vi "GeoData.vi"() -> ()   [LabVIEW 2017] (continued)
H1\n16631\t42013\tCurryville\tPA\tBlair County\tH1\n16870\t42013\tPort matilda\tPA\tBlair County\tH1\n16635\t42013\tDuncansville\tPA\tBlair County\tH1\n16613\t42013\tAshville\tPA\tBlair County\tH1\n16686\t42013\tTyrone\tPA\tBlair County\tH1\n16602\t42013\tAltoona\tPA\tBlair County\tH1\n16673\t42013\tRoaring spring\tPA\tBlair County\tH1\n16662\t42013\tMartinsburg\tPA\tBlair County\tH1\n16682\t42013\tSproul\tPA\tBlair County\tH1\n18616\t42015\tForksville\tPA\tBradford County\tH1\n18837\t42015\tRome\tPA\tBradford County\tH1\n18846\t42015\tSugar run\tPA\tBradford County\tH1\n16914\t42015\tColumbia cross roads\tPA\tBradford County\tH1\n18832\t42015\tMonroeton\tPA\tBradford County\tH1\n17765\t42015\tRoaring branch\tPA\tBradford County\tH1\n18623\t42015\tLaceyville\tPA\tBradford County\tH1\n18810\t42015\tAthens\tPA\tBradford County\tH1\n18833\t42015\tNew albany\tPA\tBradford County\tH1\n18830\t42015\tLittle meadows\tPA\tBradford County\tH1\n16926\t42015\tGranville summit\tPA\tBradford County\tH1\n18817\t42015\tEast smithfield\tPA\tBradford County\tH1\n16925\t42015\tGillett\tPA\tBradford County\tH1\n18840\t42015\tSayre\tPA\tBradford County\tH1\n18850\t42015\tUlster\tPA\tBradford County\tH1\n18814\t42015\tBurlington\tPA\tBradford County\tH1\n17735\t42015\tGrover\tPA\tBradford County\tH1\n18853\t42015\tWyalusing\tPA\tBradford County\tH1\n18854\t42015\tWysox\tPA\tBradford County\tH1\n18848\t42015\tTowanda\tPA\tBradford County\tH1\n18851\t42015\tWarren center\tPA\tBradford County\tH1\n18831\t42015\tMilan\tPA\tBradford County\tH1\n17724\t42015\tCanton\tPA\tBradford County\tH1\n18845\t42015\tStevensville\tPA\tBradford County\tH1\n16910\t42015\tAlba\tPA\tBradford County\tH1\n16936\t42015\tMillerton\tPA\tBradford County\tH1\n16947\t42015\tTroy\tPA\tBradford County\tH1\n18614\t42015\tDushore\tPA\tBradford County\tH1\n18829\t42015\tLe raysville\tPA\tBradford County\tH1\n16945\t42015\tSylvania\tPA\tBradford County\tH1\n18930\t42017\tKintnersville\tPA\tBucks County\tH1\n19006\t42017\tHuntingdon valley\tPA\tBucks County\tH1\n19047\t42017\tLanghorne\tPA\tBucks County\tH1\n19055\t42017\tLevittown\tPA\tBucks County\tH1\n18081\t42017\tSpringtown\tPA\tBucks County\tH1\n18970\t42017\tTrumbauersville\tPA\tBucks County\tH1\n18917\t42017\tDublin\tPA\tBucks County\tH1\n18931\t42017\tLahaska\tPA\tBucks County\tH1\n18968\t42017\tSpinnerstown\tPA\tBucks County\tH1\n18956\t42017\tRushland\tPA\tBucks County\tH1\n18925\t42017\tFurlong\tPA\tBucks County\tH1\n18972\t42017\tUpper black eddy\tPA\tBucks County\tH1\n19030\t42017\tFairless hills\tPA\tBucks County\tH1\n19057\t42017\tLevittown\tPA\tBucks County\tH1\n18055\t42017\tHellertown\tPA\tBucks County\tH1\n18914\t42017\tChalfont\tPA\tBucks County\tH1\n18912\t42017\tBuckingham\tPA\tBucks County\tH1\n18951\t42017\tQuakertown\tPA\tBucks County\tH1\n18964\t42017\tSouderton\tPA\tBucks County\tH1\n18942\t42017\tOttsville\tPA\tBucks County\tH1\n18977\t42017\tWashington crossing\tPA\tBucks County\tH1\n19044\t42017\tHorsham\tPA\tBucks County\tH1\n19440\t42017\tHatfield\tPA\tBucks County\tH1\n18935\t42017\tMilford square\tPA\tBucks County\tH1\n18981\t42017\tZionhill\tPA\tBucks County\tH1\n18946\t42017\tPineville\tPA\tBucks County\tH1\n18036\t42017\tCoopersburg\tPA\tBucks County\tH1\n18041\t42017\tEast greenville\tPA\tBucks County\tH1\n18077\t42017\tRiegelsville\tPA\tBucks County\tH1\n18954\t42017\tRichboro\tPA\tBucks County\tH1\n18940\t42017\tNewtown\tPA\tBucks County\tH1\n19007\t42017\tBristol\tPA\tBucks County\tH1\n19454\t42017\tNorth wales\tPA\tBucks County\tH1\n18934\t42017\tMechanicsville\tPA\tBucks County\tH1\n18933\t42017\tLumberville\tPA\tBucks County\tH1\n18915\t42017\tColmar\tPA\tBucks County\tH1\n19067\t42017\tMorrisville\tPA\tBucks County\tH1\n19053\t42017\tFeasterville trevose\tPA\tBucks County\tH1\n18949\t42017\tPlumsteadville\tPA\tBucks County\tH1\n18963\t42017\tSolebury\tPA\tBucks County\tH1\n18928\t42017\tHolicong\tPA\tBucks County\tH1\n18913\t42017\tCarversville\tPA\tBucks County\tH1\n18943\t42017\tPenns park\tPA\tBucks County\tH1\n18042\t42017\tEaston\tPA\tBucks County\tH1\n18054\t42017\tGreen lane\tPA\tBucks County\tH1\n18938\t42017\tNew hope\tPA\tBucks County\tH1\n18901\t42017\tDoylestown\tPA\tBucks County\tH1\n18929\t42017\tJamison\tPA\tBucks County\tH1\n18923\t42017\tFountainville\tPA\tBucks County\tH1\n18932\t42017\tLine lexington\tPA\tBucks County\tH1\n18974\t42017\tWarminster\tPA\tBucks County\tH1\n18960\t42017\tSellersville\tPA\tBucks County\tH1\n18976\t42017\tWarrington\tPA\tBucks County\tH1\n18947\t42017\tPipersville\tPA\tBucks County\tH1\n18962\t42017\tSilverdale\tPA\tBucks County\tH1\n19020\t42017\tBensalem\tPA\tBucks County\tH1\n19021\t42017\tCroydon\tPA\tBucks County\tH1\n19040\t42017\tHatboro\tPA\tBucks County\tH1\n18953\t42017\tRevere\tPA\tBucks County\tH1\n18911\t42017\tBlooming glen\tPA\tBucks County\tH1\n18073\t42017\tPennsburg\tPA\tBucks County\tH1\n18902\t42017\tDoylestown\tPA\tBucks County\tH1\n19056\t42017\tLevittown\tPA\tBucks County\tH1\n19058\t42017\tLevittown\tPA\tBucks County\tH1\n19054\t42017\tLevittown\tPA\tBucks County\tH1\n18955\t42017\tRichlandtown\tPA\tBucks County\tH1\n18950\t42017\tPoint pleasant\tPA\tBucks County\tH1\n18980\t42017\tWycombe\tPA\tBucks County\tH1\n18039\t42017\tDurham\tPA\tBucks County\tH1\n18944\t42017\tPerkasie\tPA\tBucks County\tH1\n18966\t42017\tSouthampton\tPA\tBucks County\tH1\n18969\t42017\tTelford\tPA\tBucks County\tH1\n18927\t42017\tHilltown\tPA\tBucks County\tH1\n18920\t42017\tErwinna\tPA\tBucks County\tH1\n18922\t42017\tForest grove\tPA\tBucks County\tH1\n18910\t42017\tBedminster\tPA\tBucks County\tH1\n18916\t42017\tDanboro\tPA\tBucks County\tH1\n18921\t42017\tFerndale\tPA\tBucks County\tH1\n16001\t42019\tButler\tPA\tButler County\tH1\n16051\t42019\tPortersville\tPA\tButler County\tH1\n16127\t42019\tGrove city\tPA\tButler County\tH1\n16059\t42019\tValencia\tPA\tButler County\tH1\n16053\t42019\tRenfrew\tPA\tButler County\tH1\n16052\t42019\tProspect\tPA\tButler County\tH1\n16041\t42019\tKarns city\tPA\tButler County\tH1\n16030\t42019\tEau claire\tPA\tButler County\tH1\n16035\t42019\tForestville\tPA\tButler County\tH1\n16024\t42019\tCallery\tPA\tButler County\tH1\n15044\t42019\tGibsonia\tPA\tButler County\tH1\n16002\t42019\tButler\tPA\tButler County\tH1\n16049\t42019\tParker\tPA\tButler County\tH1\n16038\t42019\tHarrisville\tPA\tButler County\tH1\n16040\t42019\tHilliards\tPA\tButler County\tH1\n16063\t42019\tZelienople\tPA\tButler County\tH1\n16066\t42019\tCranberry township\tPA\tButler County\tH1\n16034\t42019\tFenelton\tPA\tButler County\tH1\n16048\t42019\tNorth washington\tPA\tButler County\tH1\n16033\t42019\tEvans city\tPA\tButler County\tH1\n16373\t42019\tEmlenton\tPA\tButler County\tH1\n16050\t42019\tPetrolia\tPA\tButler County\tH1\n16029\t42019\tEast butler\tPA\tButler County\tH1\n16022\t42019\tBruin\tPA\tButler County\tH1\n16025\t42019\tChicora\tPA\tButler County\tH1\n15086\t42019\tWarrendale\tPA\tButler County\tH1\n16020\t42019\tBoyers\tPA\tButler County\tH1\n16039\t42019\tHerman\tPA\tButler County\tH1\n15065\t42019\tNatrona heights\tPA\tButler County\tH1\n16045\t42019\tLyndora\tPA\tButler County\tH1\n16023\t42019\tCabot\tPA\tButler County\tH1\n16027\t42019\tConnoquenessing\tPA\tButler County\tH1\n16046\t42019\tMars\tPA\tButler County\tH1\n16061\t42019\tWest sunbury\tPA\tButler County\tH1\n16003\t42019\tButler\tPA\tButler County\tH1\n16056\t42019\tSaxonburg\tPA\tButler County\tH1\n16057\t42019\tSlippery rock\tPA\tButler County\tH1\n16055\t42019\tSarver\tPA\tButler County\tH1\n16037\t42019\tHarmony\tPA\tButler County\tH1\n16229\t42019\tFreeport\tPA\tButler County\tH1\n15906\t42021\tJohnstown\tPA\tCambria County\tH1\n15901\t42021\tJohnstown\tPA\tCambria County\tH1\n15958\t42021\tSummerhill\tPA\tCambria County\tH1\n16639\t42021\tFallentimber\tPA\tCambria County\tH1\n15762\t42021\tNicktown\tPA\tCambria County\tH1\n15738\t42021\tEmeigh\tPA\tCambria County\tH1\n15934\t42021\tElton\tPA\tCambria County\tH1\n15930\t42021\tDunlo\tPA\tCambria County\tH1\n15714\t42021\tNorthern cambria\tPA\tCambria County\tH1\n15946\t42021\tPortage\tPA\tCambria County\tH1\n15955\t42021\tSidman\tPA\tCambria County\tH1\n16601\t42021\tAltoona\tPA\tCambria County\tH1\n15760\t42021\tMarsteller\tPA\tCambria County\tH1\n15956\t42021\tSouth fork\tPA\tCambria County\tH1\n16629\t42021\tCoupon\tPA\tCambria County\tH1\n15922\t42021\tBelsano\tPA\tCambria County\tH1\n15962\t42021\tWilmore\tPA\tCambria County\tH1\n15938\t42021\tLilly\tPA\tCambria County\tH1\n15902\t42021\tJohnstown\tPA\tCambria County\tH1\n15931\t42021\tEbensburg\tPA\tCambria County\tH1\n15940\t42021\tLoretto\tPA\tCambria County\tH1\n15957\t42021\tStrongstown\tPA\tCambria County\tH1\n16636\t42021\tDysart\tPA\tCambria County\tH1\n15927\t42021\tColver\tPA\tCambria County\tH1\n15773\t42021\tSaint benedict\tPA\tCambria County\tH1\n15904\t42021\tJohnstown\tPA\tCambria County\tH1\n15952\t42021\tSalix\tPA\tCambria County\tH1\n16641\t42021\tGallitzin\tPA\tCambria County\tH1\n16627\t42021\tCoalport\tPA\tCambria County\tH1\n16640\t42021\tFlinton\tPA\tCambria County\tH1\n16646\t42021\tHastings\tPA\tCambria County\tH1\n15961\t42021\tVintondale\tPA\tCambria County\tH1\n15921\t42021\tBeaverdale\tPA\tCambria County\tH1\n15951\t42021\tSaint michael\tPA\tCambria County\tH1\n15948\t42021\tRevloc\tPA\tCambria County\tH1\n15960\t42021\tTwin rocks\tPA\tCambria County\tH1\n15915\t42021\tJohnstown\tPA\tCambria County\tH1\n15724\t42021\tCherry tree\tPA\tCambria County\tH1\n15909\t42021\tJohnstown\tPA\tCambria County\tH1\n15943\t42021\tNanty glo\tPA\tCambria County\tH1\n15963\t42021\tWindber\tPA\tCambria County\tH1\n15722\t42021\tCarrolltown\tPA\tCambria County\tH1\n16675\t42021\tSaint boniface\tPA\tCambria County\tH1\n16624\t42021\tChest springs\tPA\tCambria County\tH1\n15907\t42021\tJohnstown\tPA\tCambria County\tH1\n16635\t42021\tDuncansville\tPA\tCambria County\tH1\n16613\t42021\tAshville\tPA\tCambria County\tH1\n16619\t42021\tBlandburg\tPA\tCambria County\tH1\n15775\t42021\tSpangler\tPA\tCambria County\tH1\n15905\t42021\tJohnstown\tPA\tCambria County\tH1\n15942\t42021\tMineral point\tPA\tCambria County\tH1\n16630\t42021\tCresson\tPA\tCambria County\tH1\n16668\t42021\tPatton\tPA\tCambria County\tH1\n15959\t42021\tTire hill\tPA\tCambria County\tH1\n15945\t42021\tParkhill\tPA\tCambria County\tH1\n15737\t42021\tElmora\tPA\tCambria County\tH1\n16644\t42021\tGlasgow\tPA\tCambria County\tH1\n15925\t42021\tCassandra\tPA\tCambria County\tH1\n15832\t42023\tDriftwood\tPA\tCameron County\tH1\n15861\t42023\tSinnamahoning\tPA\tCameron County\tH1\n16720\t42023\tAustin\tPA\tCameron County\tH1\n15834\t42023\tEmporium\tPA\tCameron County\tH1\n18211\t42025\tAndreas\tPA\tCarbon County\tH1\n18252\t42025\tTamaqua\tPA\tCarbon County\tH1\n18012\t42025\tAquashicola\tPA\tCarbon County\tH1\n18229\t42025\tJim thorpe\tPA\tCarbon County\tH1\n18254\t42025\tTresckow\tPA\tCarbon County\tH1\n18661\t42025\tWhite haven\tPA\tCarbon County\tH1\n18624\t42025\tLake harmony\tPA\tCarbon County\tH1\n18030\t42025\tBowmanstown\tPA\tCarbon County\tH1\n18053\t42025\tGermansville\tPA\tCarbon County\tH1\n18240\t42025\tNesquehoning\tPA\tCarbon County\tH1\n18333\t42025\tKresgeville\tPA\tCarbon County\tH1\n18230\t42025\tJunedale\tPA\tCarbon County\tH1\n18071\t42025\tPalmerton\tPA\tCarbon County\tH1\n18250\t42025\tSummit hill\tPA\tCarbon County\tH1\n18216\t42025\tBeaver meadows\tPA\tCarbon County\tH1\n18212\t42025\tAshfield\tPA\tCarbon County\tH1\n18232\t42025\tLansford\tPA\tCarbon County\tH1\n18244\t42025\tParryville\tPA\tCarbon County\tH1\n18201\t42025\tHazleton\tPA\tCarbon County\tH1\n18235\t42025\tLehighton\tPA\tCarbon County\tH1\n18255\t42025\tWeatherly\tPA\tCarbon County\tH1\n18237\t42025\tMcadoo\tPA\tCarbon County\tH1\n18058\t42025\tKunkletown\tPA\tCarbon County\tH1\n18210\t42025\tAlbrightsville\tPA\tCarbon County\tH1\n16820\t42027\tAaronsburg\tPA\tCentre County\tH1\n16829\t42027\tClarence\tPA\tCentre County\tH1\n16677\t42027\tSandy ridge\tPA\tCentre County\tH1\n16666\t42027\tOsceola mills\tPA\tCentre County\tH1\n16865\t42027\tPennsylvania furnace\tPA\tCentre County\tH1\n16844\t42027\tJulian\tPA\tCentre County\tH1\n16801\t42027\tState college\tPA\tCentre County\tH1\n16823\t42027\tBellefonte\tPA\tCentre County\tH1\n16866\t42027\tPhilipsburg\tPA\tCentre County\tH1\n16854\t42027\tMillheim\tPA\tCentre County\tH1\n16826\t42027\tBlanchard\tPA\tCentre County\tH1\n16804\t42027\tState college\tPA\tCentre County\tH1\n16853\t42027\tMilesburg\tPA\tCentre County\tH1\n16835\t42027\tFleming\tPA\tCentre County\tH1\n16803\t42027\tState college\tPA\tCentre County\tH1\n16827\t42027\tBoalsburg\tPA\tCentre County\tH1\n16870\t42027\tPort matilda\tPA\tCentre County\tH1\n16802\t42027\tUniversity park\tPA\tCentre County\tH1\n16872\t42027\tRebersburg\tPA\tCentre County\tH1\n16852\t42027\tMadisonburg\tPA\tCentre County\tH1\n16860\t42027\tMunson\tPA\tCentre County\tH1\n16868\t42027\tPine grove mills\tPA\tCentre County\tH1\n16856\t42027\tMingoville\tPA\tCentre County\tH1\n16686\t42027\tTyrone\tPA\tCentre County\tH1\n16828\t42027\tCentre hall\tPA\tCentre County\tH1\n16822\t42027\tBeech creek\tPA\tCentre County\tH1\n16874\t42027\tSnow shoe\tPA\tCentre County\tH1\n16845\t42027\tKarthaus\tPA\tCentre County\tH1\n16859\t42027\tMoshannon\tPA\tCentre County\tH1\n16877\t42027\tWarriors mark\tPA\tCentre County\tH1\n16851\t42027\tLemont\tPA\tCentre County\tH1\n16841\t42027\tHoward\tPA\tCentre County\tH1\n16875\t42027\tSpring mills\tPA\tCentre County\tH1\n16882\t42027\tWoodward\tPA\tCentre County\tH1\n16832\t42027\tCoburn\tPA\tCentre County\tH1\n16864\t42027\tOrviston\tPA\tCentre County\tH1\n19355\t42029\tMalvern\tPA\tChester County\tH1\n19311\t42029\tAvondale\tPA\tChester County\tH1\n19363\t42029\tOxford\tPA\tChester County\tH1\n19465\t42029\tPottstown\tPA\tChester County\tH1\n19480\t42029\tUwchland\tPA\tChester County\tH1\n19481\t42029\tValley forge\tPA\tChester County\tH1\n19357\t42029\tMendenhall\tPA\tChester County\tH1\n19432\t42029\tDevault\tPA\tChester County\tH1\n19367\t42029\tPomeroy\tPA\tChester County\tH1\n19365\t42029\tParkesburg\tPA\tChester County\tH1\n19425\t42029\tChester springs\tPA\tChester County\tH1\n19475\t42029\tSpring city\tPA\tChester County\tH1\n17536\t42029\tKirkwood\tPA\tChester County\tH1\n19354\t42029\tLyndell\tPA\tChester County\tH1\n17555\t42029\tNarvon\tPA\tChester County\tH1\n19073\t42029\tNewtown square\tPA\tChester County\tH1\n19330\t42029\tCochranville\tPA\tChester County\tH1\n19341\t42029\tExton\tPA\tChester County\tH1\n19317\t42029\tChadds ford\tPA\tChester County\tH1\n19372\t42029\tThorndale\tPA\tChester County\tH1\n19543\t42029\tMorgantown\tPA\tChester County\tH1\n19399\t42029\tSoutheastern\tPA\tChester County\tH1\n19319\t42029\tCheyney\tPA\tChester County\tH1\n19421\t42029\tBirchrunville\tPA\tChester County\tH1\n19371\t42029\tSuplee\tPA\tChester County\tH1\n17527\t42029\tGap\tPA\tChester County\tH1\n19352\t42029\tLincoln university\tPA\tChester County\tH1\n19395\t42029\tWesttown\tPA\tChester County\tH1\n19381\t42029\tWest chester\tPA\tChester County\tH1\n19460\t42029\tPhoenixville\tPA\tChester County\tH1\n19351\t42029\tLewisville\tPA\tChester County\tH1\n19347\t42029\tKemblesville\tPA\tChester County\tH1\n19366\t42029\tPocopson\tPA\tChester County\tH1\n19520\t42029\tElverson\tPA\tChester County\tH1\n19350\t42029\tLandenberg\tPA\tChester County\tH1\n19335\t42029\tDowningtown\tPA\tChester County\tH1\n19344\t42029\tHoney brook\tPA\tChester County\tH1\n19382\t42029\tWest chester\tPA\tChester County\tH1\n19464\t42029\tPottstown\tPA\tChester County\tH1\n19375\t42029\tUnionville\tPA\tChester County\tH1\n19470\t42029\tSaint peters\tPA\tChester County\tH1\n19087\t42029\tWayne\tPA\tChester County\tH1\n19348\t42029\tKennett square\tPA\tChester County\tH1\n19380\t42029\tWest chester\tPA\tChester County\tH1\n19390\t42029\tWest grove\tPA\tChester County\tH1\n19376\t42029\tWagontown\tPA\tChester County\tH1\n19316\t42029\tBrandamore\tPA\tChester County\tH1\n19320\t42029\tCoatesville\tPA\tChester County\tH1\n19333\t42029\tDevon\tPA\tChester County\tH1\n19343\t42029\tGlenmoore\tPA\tChester County\tH1\n19442\t42029\tKimberton\tPA\tChester County\tH1\n19369\t42029\tSadsburyville\tPA\tChester County\tH1\n19457\t42029\tParker ford\tPA\tChester County\tH1\n19383\t42029\tWest chester\tPA\tChester County\tH1\n19482\t42029\tValley forge\tPA\tChester County\tH1\n19374\t42029\tToughkenamon\tPA\tChester County\tH1\n19358\t42029\tModena\tPA\tChester County\tH1\n19310\t42029\tAtglen\tPA\tChester County\tH1\n19342\t42029\tGlen mills\tPA\tChester County\tH1\n19301\t42029\tPaoli\tPA\tChester County\tH1\n19312\t42029\tBerwyn\tPA\tChester County\tH1\n19362\t42029\tNottingham\tPA\tChester County\tH1\n19373\t42029\tThornton\tPA\tChester County\tH1\n19360\t42029\tNew london\tPA\tChester County\tH1\n19346\t42029\tKelton\tPA\tChester County\tH1\n19345\t42029\tImmaculata\tPA\tChester County\tH1\n19318\t42029\tChatham\tPA\tChester County\tH1\n16028\t42031\tEast brady\tPA\tClarion County\tH1\n16233\t42031\tLeeper\tPA\tClarion County\tH1\n16319\t42031\tCranberry\tPA\tClarion County\tH1\n16224\t42031\tFairmount city\tPA\tClarion County\tH1\n16364\t42031\tVenus\tPA\tClarion County\tH1\n16326\t42031\tFryburg\tPA\tClarion County\tH1\n16331\t42031\tKossuth\tPA\tClarion County\tH1\n16225\t42031\tFisher\tPA\tClarion County\tH1\n16221\t42031\tCurllsville\tPA\tClarion County\tH1\n16242\t42031\tNew bethlehem\tPA\tClarion County\tH1\n16232\t42031\tKnox\tPA\tClarion County\tH1\n16248\t42031\tRimersburg\tPA\tClarion County\tH1\n16235\t42031\tLucinda\tPA\tClarion County\tH1\n16334\t42031\tMarble\tPA\tClarion County\tH1\n16361\t42031\tTylersburg\tPA\tClarion County\tH1\n16049\t42031\tParker\tPA\tClarion County\tH1\n16217\t42031\tCooksburg\tPA\tClarion County\tH1\n16353\t42031\tTionesta\tPA\tClarion County\tH1\n16332\t42031\tLickingville\tPA\tClarion County\tH1\n16054\t42031\tSaint petersburg\tPA\tClarion County\tH1\n16223\t42031\tDistant\tPA\tClarion County\tH1\n16213\t42031\tCallensburg\tPA\tClarion County\tH1\n15829\t42031\tCorsica\tPA\tClarion County\tH1\n16373\t42031\tEmlenton\tPA\tClarion County\tH1\n16036\t42031\tFoxburg\tPA\tClarion County\tH1\n16214\t42031\tClarion\tPA\tClarion County\tH1\n16258\t42031\tStrattanville\tPA\tClarion County\tH1\n16220\t42031\tCrown\tPA\tClarion County\tH1\n16240\t42031\tMayport\tPA\tClarion County\tH1\n16230\t42031\tHawthorn\tPA\tClarion County\tH1\n16058\t42031\tTurkey city\tPA\tClarion County\tH1\n16375\t42031\tLamartine\tPA\tClarion County\tH1\n16234\t42031\tLimestone\tPA\tClarion County\tH1\n15860\t42031\tSigel\tPA\tClarion County\tH1\n16260\t42031\tVowinckel\tPA\tClarion County\tH1\n16239\t42031\tMarienville\tPA\tClarion County\tH1\n15864\t42031\tSummerville\tPA\tClarion County\tH1\n16254\t42031\tShippenville\tPA\tClarion County\tH1\n16255\t42031\tSligo\tPA\tClarion County\tH1\n15801\t42033\tDu bois\tPA\tClearfield County\tH1\n15840\t42033\tFalls creek\tPA\tClearfield County\tH1\n16639\t42033\tFallentimber\tPA\tClearfield County\tH1\n16661\t42033\tMadera\tPA\tClearfield County\tH1\n16836\t42033\tFrenchville\tPA\tClearfield County\tH1\n16843\t42033\tHyde\tPA\tClearfield County\tH1\n16850\t42033\tLecontes mills\tPA\tClearfield County\tH1\n16663\t42033\tMorann\tPA\tClearfield County\tH1\n15824\t42033\tBrockway\tPA\tClearfield County\tH1\n16666\t42033\tOsceola mills\tPA\tClearfield County\tH1\n16863\t42033\tOlanta\tPA\tClearfield County\tH1\n16881\t42033\tWoodland\tPA\tClearfield County\tH1\n16858\t42033\tMorrisdale\tPA\tClearfield County\tH1\n16821\t42033\tAllport\tPA\tClearfield County\tH1\n16681\t42033\tSmokerun\tPA\tClearfield County\tH1\n16847\t42033\tKylertown\tPA\tClearfield County\tH1\n15721\t42033\tBurnside\tPA\tClearfield County\tH1\n15851\t42033\tReynoldsville\tPA\tClearfield County\tH1\n15865\t42033\tSykesville\tPA\tClearfield County\tH1\n15856\t42033\tRockton\tPA\tClearfield County\tH1\n16837\t42033\tGlen richey\tPA\tClearfield County\tH1\n16879\t42033\tWinburne\tPA\tClearfield County\tH1\n16671\t42033\tRamey\tPA\tClearfield County\tH1\n15767\t42033\tPunxsutawney\tPA\tClearfield County\tH1\n15823\t42033\tBrockport\tPA\tClearfield County\tH1\n15848\t42033\tLuthersburg\tPA\tClearfield County\tH1\n16651\t42033\tHoutzdale\tPA\tClearfield County\tH1\n16866\t42033\tPhilipsburg\tPA\tClearfield County\tH1\n16839\t42033\tGrassflat\tPA\tClearfield County\tH1\n16840\t42033\tHawk run\tPA\tClearfield County\tH1\n16825\t42033\tBigler\tPA\tClearfield County\tH1\n16849\t42033\tLanse\tPA\tClearfield County\tH1\n15757\t42033\tMahaffey\tPA\tClearfield County\tH1\n15753\t42033\tLa jose\tPA\tClearfield County\tH1\n16627\t42033\tCoalport\tPA\tClearfield County\tH1\n16640\t42033\tFlinton\tPA\tClearfield County\tH1\n16646\t42033\tHastings\tPA\tClearfield County\tH1\n16876\t42033\tWallaceton\tPA\tClearfield County\tH1\n15866\t42033\tTroutville\tPA\tClearfield County\tH1\n16855\t42033\tMineral springs\tPA\tClearfield County\tH1\n15742\t42033\tGlen campbell\tPA\tClearfield County\tH1\n15724\t42033\tCherry tree\tPA\tClearfield County\tH1\n16692\t42033\tWestover\tPA\tClearfield County\tH1\n16645\t42033\tGlen hope\tPA\tClearfield County\tH1\n16616\t42033\tBeccaria\tPA\tClearfield County\tH1\n16871\t42033\tPottersdale\tPA\tClearfield County\tH1\n16860\t42033\tMunson\tPA\tClearfield County\tH1\n16620\t42033\tBrisbin\tPA\tClearfield County\tH1\n16656\t42033\tIrvona\tPA\tClearfield County\tH1\n16830\t42033\tClearfield\tPA\tClearfield County\tH1\n16878\t42033\tWest decatur\tPA\tClearfield County\tH1\n16845\t42033\tKarthaus\tPA\tClearfield County\tH1\n16861\t42033\tNew millport\tPA\tClearfield County\tH1\n16680\t42033\tSmithmill\tPA\tClearfield County\tH1\n15849\t42033\tPenfield\tPA\tClearfield County\tH1\n16833\t42033\tCurwensville\tPA\tClearfield County\tH1\n16838\t42033\tGrampian\tPA\tClearfield County\tH1\n16873\t42033\tShawville\tPA\tClearfield County\tH1\n16834\t42033\tDrifting\tPA\tClearfield County\tH1\n17764\t42035\tRenovo\tPA\tClinton County\tH1\n17745\t42035\tLock haven\tPA\tClinton County\tH1\n17760\t42035\tNorth bend\tPA\tClinton County\tH1\n17751\t42035\tMill hall\tPA\tClinton County\tH1\n16848\t42035\tLamar\tPA\tClinton County\tH1\n17779\t42035\tWoolrich\tPA\tClinton County\tH1\n16871\t42035\tPottersdale\tPA\tClinton County\tH1\n17750\t42035\tMackeyville\tPA\tClinton County\tH1\n17748\t42035\tMc elhattan\tPA\tClinton County\tH1\n16822\t42035\tBeech creek\tPA\tClinton County\tH1\n16845\t42035\tKarthaus\tPA\tClinton County\tH1\n17747\t42035\tLoganton\tPA\tClinton County\tH1\n17729\t42035\tCross fork\tPA\tClinton County\tH1\n16841\t42035\tHoward\tPA\tClinton County\tH1\n17721\t42035\tAvis\tPA\tClinton County\tH1\n17740\t42035\tJersey shore\tPA\tClinton County\tH1\n17778\t42035\tWestport\tPA\tClinton County\tH1\n16864\t42035\tOrviston\tPA\tClinton County\tH1\n17726\t42035\tCastanea\tPA\tClinton County\tH1\n17814\t42037\tBenton\tPA\tColumbia County\tH1\n17859\t42037\tOrangeville\tPA\tColumbia County\tH1\n17921\t42037\tAshland\tPA\tColumbia County\tH1\n18655\t42037\tShickshinny\tPA\tColumbia County\tH1\n18635\t42037\tNescopeck\tPA\tColumbia County\tH1\n17878\t42037\tStillwater\tPA\tColumbia County\tH1\n17756\t42037\tMuncy\tPA\tColumbia County\tH1\n17772\t42037\tTurbotville\tPA\tColumbia County\tH1\n17824\t42037\tElysburg\tPA\tColumbia County\tH1\n18249\t42037\tSugarloaf\tPA\tColumbia County\tH1\n17967\t42037\tRingtown\tPA\tColumbia County\tH1\n17888\t42037\tWilburton\tPA\tColumbia County\tH1\n17821\t42037\tDanville\tPA\tColumbia County\tH1\n17815\t42037\tBloomsburg\tPA\tColumbia County\tH1\n17847\t42037\tMilton\tPA\tColumbia County\tH1\n17920\t42037\tAristes\tPA\tColumbia County\tH1\n18603\t42037\tBerwick\tPA\tColumbia County\tH1\n17820\t42037\tCatawissa\tPA\tColumbia County\tH1\n17858\t42037\tNumidia\tPA\tColumbia County\tH1\n17846\t42037\tMillville\tPA\tColumbia County\tH1\n17774\t42037\tUnityville\tPA\tColumbia County\tH1\n17985\t42037\tZion grove\tPA\tColumbia County\tH1\n18631\t42037\tMifflinville\tPA\tColumbia County\tH1\n16134\t42039\tJamestown\tPA\tCrawford County\tH1\n16335\t42039\tMeadville\tPA\tCrawford County\tH1\n16435\t42039\tSpringboro\tPA\tCrawford County\tH1\n16424\t42039\tLinesville\tPA\tCrawford County\tH1\n16131\t42039\tHartstown\tPA\tCrawford County\tH1\n16314\t42039\tCochranton\tPA\tCrawford County\tH1\n16403\t42039\tCambridge springs\tPA\tCrawford County\tH1\n16438\t42039\tUnion city\tPA\tCrawford County\tH1\n16125\t42039\tGreenville\tPA\tCrawford County\tH1\n16407\t42039\tCorry\tPA\tCrawford County\tH1\n16111\t42039\tAtlantic\tPA\tCrawford County\tH1\n16360\t42039\tTownville\tPA\tCrawford County\tH1\n16440\t42039\tVenango\tPA\tCrawford County\tH1\n16388\t42039\tMeadville\tPA\tCrawford County\tH1\n16422\t42039\tHarmonsburg\tPA\tCrawford County\tH1\n16354\t42039\tTitusville\tPA\tCrawford County\tH1\n16328\t42039\tHydetown\tPA\tCrawford County\tH1\n16406\t42039\tConneautville\tPA\tCrawford County\tH1\n16317\t42039\tCooperstown\tPA\tCrawford County\tH1\n16110\t42039\tAdamsville\tPA\tCrawford County\tH1\n16130\t42039\tHadley\tPA\tCrawford County\tH1\n16327\t42039\tGuys mills\tPA\tCrawford County\tH1\n16316\t42039\tConneaut lake\tPA\tCrawford County\tH1\n16434\t42039\tSpartansburg\tPA\tCrawford County\tH1\n16441\t42039\tWaterford\tPA\tCrawford County\tH1\n16362\t42039\tUtica\tPA\tCrawford County\tH1\n16412\t42039\tEdinboro\tPA\tCrawford County\tH1\n16433\t42039\tSaegertown\tPA\tCrawford County\tH1\n16401\t42039\tAlbion\tPA\tCrawford County\tH1\n16404\t42039\tCenterville\tPA\tCrawford County\tH1\n16420\t42039\tGrand valley\tPA\tCrawford County\tH1\n17007\t42041\tBoiling springs\tPA\tCumberland County\tH1\n17025\t42041\tEnola\tPA\tCumberland County\tH1\n17050\t42041\tMechanicsburg\tPA\tCumberland County\tH1\n17090\t42041\tShermans dale\tPA\tCumberland County\tH1\n17065\t42041\tMount holly springs\tPA\tCumberland County\tH1\n17307\t42041\tBiglerville\tPA\tCumberland County\tH1\n17013\t42041\tCarlisle\tPA\tCumberland County\tH1\n17324\t42041\tGardners\tPA\tCumberland County\tH1\n17001\t42041\tCamp hill\tPA\tCumberland County\tH1\n17015\t42041\tCarlisle\tPA\tCumberland County\tH1\n17043\t42041\tLemoyne\tPA\tCumberland County\tH1\n17240\t42041\tNewburg\tPA\tCumberland County\tH1\n17053\t42041\tMarysville\tPA\tCumberland County\tH1\n17093\t42041\tSummerdale\tPA\tCumberland County\tH1\n17072\t42041\tNew kingstown\tPA\tCumberland County\tH1\n17027\t42041\tGrantham\tPA\tCumberland County\tH1\n17019\t42041\tDillsburg\tPA\tCumberland County\tH1\n17266\t42041\tWalnut bottom\tPA\tCumberland County\tH1\n17011\t42041\tCamp hill\tPA\tCumberland County\tH1\n17070\t42041\tNew cumberland\tPA\tCumberland County\tH1\n17081\t42041\tPlainfield\tPA\tCumberland County\tH1\n17089\t42041\tCamp hill\tPA\tCumberland County\tH1\n17055\t42041\tMechanicsburg\tPA\tCumberland County\tH1\n17241\t42041\tNewville\tPA\tCumberland County\tH1\n17257\t42041\tShippensburg\tPA\tCumberland County\tH1\n17033\t42043\tHershey\tPA\tDauphin County\tH1\n17036\t42043\tHummelstown\tPA\tDauphin County\tH1\n17111\t42043\tHarrisburg\tPA\tDauphin County\tH1\n17120\t42043\tHarrisburg\tPA\tDauphin County\tH1\n17129\t42043\tHarrisburg\tPA\tDauphin County\tH1\n17005\t42043\tBerrysburg\tPA\tDauphin County\tH1\n17023\t42043\tElizabethville\tPA\tDauphin County\tH1\n17028\t42043\tGrantville\tPA\tDauphin County\tH1\n17101\t42043\tHarrisburg\tPA\tDauphin County\tH1\n17980\t42043\tTower city\tPA\tDauphin County\tH1\n17105\t42043\tHarrisburg\tPA\tDauphin County\tH1\n17978\t42043\tSpring glen\tPA\tDauphin County\tH1\n17048\t42043\tLykens\tPA\tDauphin County\tH1\n17078\t42043\tPalmyra\tPA\tDauphin County\tH1\n17061\t42043\tMillersburg\tPA\tDauphin County\tH1\n17034\t42043\tHighspire\tPA\tDauphin County\tH1\n17017\t42043\tDalmatia\tPA\tDauphin County\tH1\n17030\t42043\tGratz\tPA\tDauphin County\tH1\n17107\t42043\tHarrisburg\tPA\tDauphin County\tH1\n17108\t42043\tHarrisburg\tPA\tDauphin County\tH1\n17128\t42043\tHarrisburg\tPA\tDauphin County\tH1\n17123\t42043\tHarrisburg\tPA\tDauphin County\tH1\n17057\t42043\tMiddletown\tPA\tDauphin County\tH1\n17109\t42043\tHarrisburg\tPA\tDauphin County\tH1\n17127\t42043\tHarrisburg\tPA\tDauphin County\tH1\n17130\t42043\tHarrisburg\tPA\tDauphin County\tH1\n17102\t42043\tHarrisburg\tPA\tDauphin County\tH1\n17106\t42043\tHarrisburg\tPA\tDauphin County\tH1\n17177\t42043\tHarrisburg\tPA\tDauphin County\tH1\n17122\t42043\tHarrisburg\tPA\tDauphin County\tH1\n17103\t42043\tHarrisburg\tPA\tDauphin County\tH1\n19405\t42043\tBridgeport\tPA\tDauphin County\tH1\n17018\t42043\tDauphin\tPA\tDauphin County\tH1\n17032\t42043\tHalifax\tPA\tDauphin County\tH1\n17110\t42043\tHarrisburg\tPA\tDauphin County\tH1\n17098\t42043\tWilliamstown\tPA\tDauphin County\tH1\n17121\t42043\tHarrisburg\tPA\tDauphin County\tH1\n17080\t42043\tPillow\tPA\tDauphin County\tH1\n17125\t42043\tHarrisburg\tPA\tDauphin County\tH1\n17126\t42043\tHarrisburg\tPA\tDauphin County\tH1\n17022\t42043\tElizabethtown\tPA\tDauphin County\tH1\n17020\t42043\tDuncannon\tPA\tDauphin County\tH1\n17104\t42043\tHarrisburg\tPA\tDauphin County\tH1\n17112\t42043\tHarrisburg\tPA\tDauphin County\tH1\n17113\t42043\tHarrisburg\tPA\tDauphin County\tH1\n17097\t42043\tWiconisco\tPA\tDauphin County\tH1\n17124\t42043\tHarrisburg\tPA\tDauphin County\tH1\n19064\t42045\tSpringfield\tPA\tDelaware County\tH1\n19081\t42045\tSwarthmore\tPA\tDelaware County\tH1\n19076\t42045\tProspect park\tPA\tDelaware County\tH1\n19018\t42045\tClifton heights\tPA\tDelaware County\tH1\n19023\t42045\tDarby\tPA\tDelaware County\tH1\n19074\t42045\tNorwood\tPA\tDelaware County\tH1\n19083\t42045\tHavertown\tPA\tDelaware County\tH1\n19082\t42045\tUpper darby\tPA\tDelaware County\tH1\n19010\t42045\tBryn mawr\tPA\tDelaware County\tH1\n19022\t42045\tCrum lynne\tPA\tDelaware County\tH1\n19063\t42045\tMedia\tPA\tDelaware County\tH1\n19073\t42045\tNewtown square\tPA\tDelaware County\tH1\n19317\t42045\tChadds ford\tPA\tDelaware County\tH1\n19113\t42045\tPhiladelphia\tPA\tDelaware County\tH1\n19028\t42045\tEdgemont\tPA\tDelaware County\tH1\n19319\t42045\tCheyney\tPA\tDelaware County\tH1\n19013\t42045\tChester\tPA\tDelaware County\tH1\n19050\t42045\tLansdowne\tPA\tDelaware County\tH1\n19079\t42045\tSharon hill\tPA\tDelaware County\tH1\n19094\t42045\tWoodlyn\tPA\tDelaware County\tH1\n19070\t42045\tMorton\tPA\tDelaware County\tH1\n19043\t42045\tHolmes\tPA\tDelaware County\tH1\n19339\t42045\tConcordville\tPA\tDelaware County\tH1\n19003\t42045\tArdmore\tPA\tDelaware County\tH1\n19026\t42045\tDrexel hill\tPA\tDelaware County\tH1\n19029\t42045\tEssington\tPA\tDelaware County\tH1\n19033\t42045\tFolsom\tPA\tDelaware County\tH1\n19096\t42045\tWynnewood\tPA\tDelaware County\tH1\n19382\t42045\tWest chester\tPA\tDelaware County\tH1\n19091\t42045\tMedia\tPA\tDelaware County\tH1\n19052\t42045\tLenni\tPA\tDelaware County\tH1\n19036\t42045\tGlenolden\tPA\tDelaware County\tH1\n19078\t42045\tRidley park\tPA\tDelaware County\tH1\n19087\t42045\tWayne\tPA\tDelaware County\tH1\n19032\t42045\tFolcroft\tPA\tDelaware County\tH1\n19060\t42045\tGarnet valley\tPA\tDelaware County\tH1\n19086\t42045\tWallingford\tPA\tDelaware County\tH1\n19333\t42045\tDevon\tPA\tDelaware County\tH1\n19016\t42045\tChester\tPA\tDelaware County\tH1\n19331\t42045\tConcordville\tPA\tDelaware County\tH1\n19039\t42045\tGradyville\tPA\tDelaware County\tH1\n19014\t42045\tAston\tPA\tDelaware County\tH1\n19015\t42045\tBrookhaven\tPA\tDelaware County\tH1\n19008\t42045\tBroomall\tPA\tDelaware County\tH1\n19061\t42045\tMarcus hook\tPA\tDelaware County\tH1\n19085\t42045\tVillanova\tPA\tDelaware County\tH1\n19153\t42045\tPhiladelphia\tPA\tDelaware County\tH1\n19342\t42045\tGlen mills\tPA\tDelaware County\tH1\n19312\t42045\tBerwyn\tPA\tDelaware County\tH1\n19041\t42045\tHaverford\tPA\tDelaware County\tH1\n19017\t42045\tChester heights\tPA\tDelaware County\tH1\n19373\t42045\tThornton\tPA\tDelaware County\tH1\n15821\t42047\tBenezett\tPA\tElk County\tH1\n15828\t42047\tClarington\tPA\tElk County\tH1\n15822\t42047\tBrandy camp\tPA\tElk County\tH1\n15845\t42047\tJohnsonburg\tPA\tElk County\tH1\n15853\t42047\tRidgway\tPA\tElk County\tH1\n15824\t42047\tBrockway\tPA\tElk County\tH1\n15831\t42047\tDagus mines\tPA\tElk County\tH1\n15870\t42047\tWilcox\tPA\tElk County\tH1\n15823\t42047\tBrockport\tPA\tElk County\tH1\n15832\t42047\tDriftwood\tPA\tElk County\tH1\n16735\t42047\tKane\tPA\tElk County\tH1\n15846\t42047\tKersey\tPA\tElk County\tH1\n15827\t42047\tByrnedale\tPA\tElk County\tH1\n15857\t42047\tSaint marys\tPA\tElk County\tH1\n16734\t42047\tJames city\tPA\tElk County\tH1\n15860\t42047\tSigel\tPA\tElk County\tH1\n15868\t42047\tWeedville\tPA\tElk County\tH1\n15834\t42047\tEmporium\tPA\tElk County\tH1\n15841\t42047\tForce\tPA\tElk County\tH1\n16435\t42049\tSpringboro\tPA\tErie County\tH1\n16505\t42049\tErie\tPA\tErie County\tH1\n16443\t42049\tWest springfield\tPA\tErie County\tH1\n16511\t42049\tErie\tPA\tErie County\tH1\n16514\t42049\tErie\tPA\tErie County\tH1\n16423\t42049\tLake city\tPA\tErie County\tH1\n16428\t42049\tNorth east\tPA\tErie County\tH1\n16403\t42049\tCambridge springs\tPA\tErie County\tH1\n16438\t42049\tUnion city\tPA\tErie County\tH1\n16503\t42049\tErie\tPA\tErie County\tH1\n16550\t42049\tErie\tPA\tErie County\tH1\n16544\t42049\tErie\tPA\tErie County\tH1\n16546\t42049\tErie\tPA\tErie County\tH1\n16407\t42049\tCorry\tPA\tErie County\tH1\n16421\t42049\tHarborcreek\tPA\tErie County\tH1\n16512\t42049\tErie\tPA\tErie County\tH1\n16534\t42049\tErie\tPA\tErie County\tH1\n16430\t42049\tNorth springfield\tPA\tErie County\tH1\n16444\t42049\tEdinboro\tPA\tErie County\tH1\n16427\t42049\tMill village\tPA\tErie County\tH1\n16415\t42049\tFairview\tPA\tErie County\tH1\n16410\t42049\tCranesville\tPA\tErie County\tH1\n16504\t42049\tErie\tPA\tErie County\tH1\n16507\t42049\tErie\tPA\tErie County\tH1\n16541\t42049\tErie\tPA\tErie County\tH1\n16563\t42049\tErie\tPA\tErie County\tH1\n16515\t42049\tErie\tPA\tErie County\tH1\n16509\t42049\tErie\tPA\tErie County\tH1\n16442\t42049\tWattsburg\tPA\tErie County\tH1\n16506\t42049\tErie\tPA\tErie County\tH1\n16475\t42049\tAlbion\tPA\tErie County\tH1\n16413\t42049\tElgin\tPA\tErie County\tH1\n16434\t42049\tSpartansburg\tPA\tErie County\tH1\n16441\t42049\tWaterford\tPA\tErie County\tH1\n16502\t42049\tErie\tPA\tErie County\tH1\n16565\t42049\tErie\tPA\tErie County\tH1\n16411\t42049\tEast springfield\tPA\tErie County\tH1\n16530\t42049\tErie\tPA\tErie County\tH1\n16412\t42049\tEdinboro\tPA\tErie County\tH1\n16401\t42049\tAlbion\tPA\tErie County\tH1\n16417\t42049\tGirard\tPA\tErie County\tH1\n16426\t42049\tMc kean\tPA\tErie County\tH1\n16510\t42049\tErie\tPA\tErie County\tH1\n16508\t42049\tErie\tPA\tErie County\tH1\n16501\t42049\tErie\tPA\tErie County\tH1\n15442\t42051\tGrindstone\tPA\tFayette County\tH1\n15461\t42051\tMasontown\tPA\tFayette County\tH1\n15492\t42051\tWickhaven\tPA\tFayette County\tH1\n15622\t42051\tChampion\tPA\tFayette County\tH1\n15490\t42051\tWhite\tPA\tFayette County\tH1\n15416\t42051\tBrownfield\tPA\tFayette County\tH1\n15462\t42051\tMelcroft\tPA\tFayette County\tH1\n15476\t42051\tRonco\tPA\tFayette County\tH1\n15475\t42051\tRepublic\tPA\tFayette County\tH1\n15482\t42051\tStar junction\tPA\tFayette County\tH1\n15012\t42051\tBelle vernon\tPA\tFayette County\tH1\n15437\t42051\tFarmington\tPA\tFayette County\tH1\n15469\t42051\tNormalville\tPA\tFayette County\tH1\n15444\t42051\tHiller\tPA\tFayette County\tH1\n15433\t42051\tEast millsboro\tPA\tFayette County\tH1\n15454\t42051\tLeckrone\tPA\tFayette County\tH1\n15439\t42051\tGans\tPA\tFayette County\tH1\n15428\t42051\tDawson\tPA\tFayette County\tH1\n15557\t42051\tRockwood\tPA\tFayette County\tH1\n15467\t42051\tNew geneva\tPA\tFayette County\tH1\n15420\t42051\tCardale\tPA\tFayette County\tH1\n15455\t42051\tLeisenring\tPA\tFayette County\tH1\n15464\t42051\tMill run\tPA\tFayette County\tH1\n15631\t42051\tEverson\tPA\tFayette County\tH1\n15466\t42051\tNewell\tPA\tFayette County\tH1\n15421\t42051\tChalk hill\tPA\tFayette County\tH1\n15401\t42051\tUniontown\tPA\tFayette County\tH1\n15417\t42051\tBrownsville\tPA\tFayette County\tH1\n15425\t42051\tConnellsville\tPA\tFayette County\tH1\n15478\t42051\tSmithfield\tPA\tFayette County\tH1\n15610\t42051\tAcme\tPA\tFayette County\tH1\n15458\t42051\tMc clellandtown\tPA\tFayette County\tH1\n15435\t42051\tFairbank\tPA\tFayette County\tH1\n15446\t42051\tIndian head\tPA\tFayette County\tH1\n15410\t42051\tAdah\tPA\tFayette County\tH1\n15460\t42051\tMartin\tPA\tFayette County\tH1\n15484\t42051\tUledi\tPA\tFayette County\tH1\n15422\t42051\tChestnut ridge\tPA\tFayette County\tH1\n15443\t42051\tHibbs\tPA\tFayette County\tH1\n15320\t42051\tCarmichaels\tPA\tFayette County\tH1\n15486\t42051\tVanderbilt\tPA\tFayette County\tH1\n15431\t42051\tDunbar\tPA\tFayette County\tH1\n15459\t42051\tMarkleysburg\tPA\tFayette County\tH1\n15473\t42051\tPerryopolis\tPA\tFayette County\tH1\n15451\t42051\tLake lynn\tPA\tFayette County\tH1\n15488\t42051\tWaltersburg\tPA\tFayette County\tH1\n15465\t42051\tMount braddock\tPA\tFayette County\tH1\n15489\t42051\tWest leisenring\tPA\tFayette County\tH1\n15472\t42051\tOliver\tPA\tFayette County\tH1\n15449\t42051\tKeisterville\tPA\tFayette County\tH1\n15474\t42051\tPoint marion\tPA\tFayette County\tH1\n15470\t42051\tOhiopyle\tPA\tFayette County\tH1\n15666\t42051\tMount pleasant\tPA\tFayette County\tH1\n15683\t42051\tScottdale\tPA\tFayette County\tH1\n15480\t42051\tSmock\tPA\tFayette County\tH1\n15430\t42051\tDickerson run\tPA\tFayette County\tH1\n15445\t42051\tHopwood\tPA\tFayette County\tH1\n15413\t42051\tAllison\tPA\tFayette County\tH1\n15456\t42051\tLemont furnace\tPA\tFayette County\tH1\n15438\t42051\tFayette city\tPA\tFayette County\tH1\n15468\t42051\tNew salem\tPA\tFayette County\tH1\n15424\t42051\tConfluence\tPA\tFayette County\tH1\n15436\t42051\tFairchance\tPA\tFayette County\tH1\n15440\t42051\tGibbon glade\tPA\tFayette County\tH1\n15450\t42051\tLa belle\tPA\tFayette County\tH1\n15447\t42051\tIsabella\tPA\tFayette County\tH1\n15463\t42051\tMerrittstown\tPA\tFayette County\tH1\n15415\t42051\tBrier hill\tPA\tFayette County\tH1\n15828\t42053\tClarington\tPA\tForest County\tH1\n16321\t42053\tEast hickory\tPA\tForest County\tH1\n16217\t42053\tCooksburg\tPA\tForest County\tH1\n16341\t42053\tPleasantville\tPA\tForest County\tH1\n16353\t42053\tTionesta\tPA\tForest County\tH1\n16351\t42053\tTidioute\tPA\tForest County\tH1\n16347\t42053\tSheffield\tPA\tForest County\tH1\n16260\t42053\tVowinckel\tPA\tForest County\tH1\n16239\t42053\tMarienville\tPA\tForest County\tH1\n16322\t42053\tEndeavor\tPA\tForest County\tH1\n16370\t42053\tWest hickory\tPA\tForest County\tH1\n17214\t42055\tBlue ridge summit\tPA\tFranklin County\tH1\n17210\t42055\tAmberson\tPA\tFranklin County\tH1\n17222\t42055\tFayetteville\tPA\tFranklin County\tH1\n17236\t42055\tMercersburg\tPA\tFranklin County\tH1\n17265\t42055\tUpperstrasburg\tPA\tFranklin County\tH1\n17232\t42055\tLurgan\tPA\tFranklin County\tH1\n17021\t42055\tEast waterford\tPA\tFranklin County\tH1\n17224\t42055\tFort loudon\tPA\tFranklin County\tH1\n17219\t42055\tDoylesburg\tPA\tFranklin County\tH1\n17268\t42055\tWaynesboro\tPA\tFranklin County\tH1\n17252\t42055\tSaint thomas\tPA\tFranklin County\tH1\n17250\t42055\tRouzerville\tPA\tFranklin County\tH1\n17246\t42055\tPleasant hall\tPA\tFranklin County\tH1\n17231\t42055\tLemasters\tPA\tFranklin County\tH1\n17272\t42055\tZullinger\tPA\tFranklin County\tH1\n17247\t42055\tQuincy\tPA\tFranklin County\tH1\n17240\t42055\tNewburg\tPA\tFranklin County\tH1\n17235\t42055\tMarion\tPA\tFranklin County\tH1\n17217\t42055\tConcord\tPA\tFranklin County\tH1\n17233\t42055\tMc connellsburg\tPA\tFranklin County\tH1\n17221\t42055\tFannettsburg\tPA\tFranklin County\tH1\n17256\t42055\tShady grove\tPA\tFranklin County\tH1\n17244\t42055\tOrrstown\tPA\tFranklin County\tH1\n17262\t42055\tSpring run\tPA\tFranklin County\tH1\n17271\t42055\tWillow hill\tPA\tFranklin County\tH1\n17202\t42055\tChambersburg\tPA\tFranklin County\tH1\n17201\t42055\tChambersburg\tPA\tFranklin County\tH1\n17237\t42055\tMont alto\tPA\tFranklin County\tH1\n17220\t42055\tDry run\tPA\tFranklin County\tH1\n17254\t42055\tScotland\tPA\tFranklin County\t
